vi "Get Flow Rate.vi"(8 "error in":errorcluster, 9 "GEN-SYS Subunit":T1, 11 "Owlstone GEN-SYS in":refnum<class "Owlstone GEN-SYS.lvclass">) -> (0 "error out":errorcluster, 1 "Flow Setpoint":sgl, 2 "Flow Value":sgl, 3 "Owlstone GEN-SYS out":refnum<class "Owlstone GEN-SYS.lvclass">)   [LabVIEW 2011, in "Owlstone GEN-SYS.lvclass"]
uses:
  Owlstone GEN-SYS.lvclass
  GEN-SYS subunit.ctl
  Owlstone GEN-SYS.lvclass/Owlstone GEN-SYS.ctl
  <instrlib>/Eurotherm 32xx Series/Eurotherm 32xx Series.lvlib
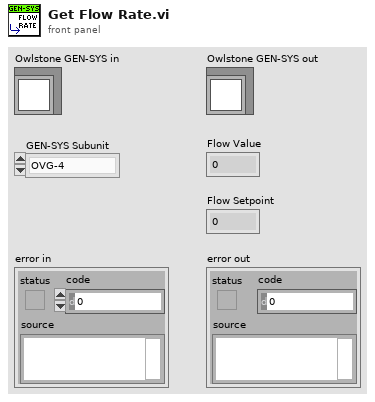
[diagram p1: front panel]
types:
  T1 = typedef "Owlstone GEN-SYS.lvclass/GEN-SYS subunit.ctl" = enum16{"OVG-4", "OHG-4", "OFC-1"}
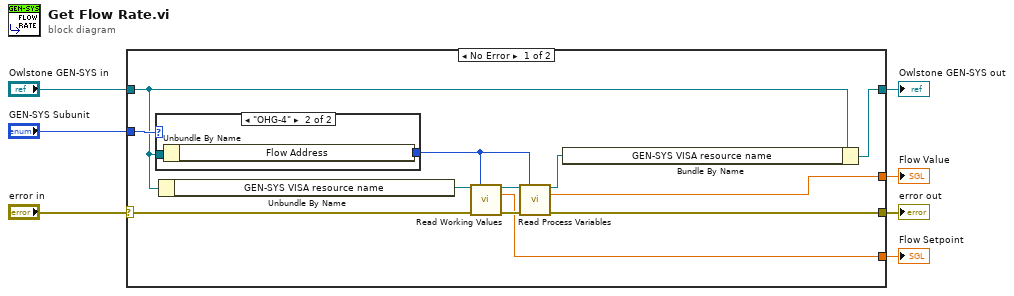
[diagram p0: block diagram]
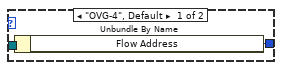
[diagram p2: hidden frame]
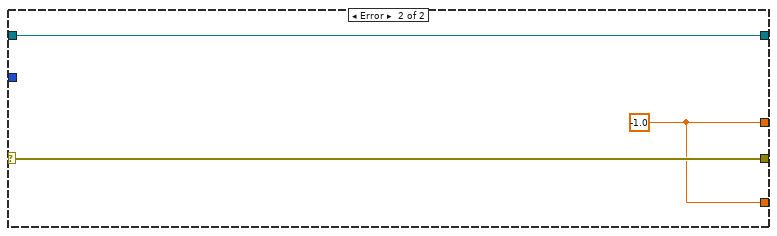
[diagram p3: hidden frame]
diagram:
  n1 = case shown="No Error" "error in" {
    selector: "error in" -> [w8 w26]
    tunnel: [w19 w25] -> w7
    tunnel: [w15 w26] -> w6
    tunnel: [w14 w24] -> w5
    tunnel: [w13 w24] -> w4
    tunnel: "GEN-SYS Subunit" -> [w11 _]
    tunnel: "Owlstone GEN-SYS in" -> [w10 w25]
    frame No Error {
      n2 = case shown="\"OHG-4\"" w11 {
        tunnel: w10 -> [w21 w23]
        tunnel: [w20 w22] -> w9
        frame "OVG-4", Default {
          n3 = Unbundle By Name(w21) -> ("Flow Address"=w20:u8)
        }
        frame "OHG-4" {
          n4 = Unbundle By Name(w23) -> ("Flow Address"=w22:u8)
        }
      }
      n5 = Unbundle By Name(w10) -> ("GEN-SYS VISA resource name"=w12:refnum<visa-resource-name>)
      n6 = call <instrlib>:"Read Working Values.vi"("VISA resource name"=w12, "Unit Address (1)"=w9, "error in (no error)"=w8) -> ("VISA resource name out"=w16:refnum<visa-resource-name>, "Working Setpoint (0)"=w14:sgl, "error out"=w17:errorcluster)  [unwired: 9 in, 1 out]
      n7 = call <instrlib>:"Read Process Variables.vi"("VISA resource name"=w16, "Unit Address (1)"=w9, "error in (no error)"=w17) -> ("VISA resource name out"=w18:refnum<visa-resource-name>, "Process Value"=w13:sgl, "error out"=w15:errorcluster)  [unwired: 9 in, 1 out]
      n8 = Bundle By Name(cluster=w10, "GEN-SYS VISA resource name"=w18) -> (w19:refnum<class "Owlstone GEN-SYS.lvclass">)
    }
    frame Error {
      w24 = sgl -1.0 ("Process Value")
    }
  }
  "Owlstone GEN-SYS out" <- w7
  "error out" <- w6
  "Flow Setpoint" <- w5
  "Flow Value" <- w4
